vi "ClassNameCompare1.vi"(10 "NodeClass":string, 11 "classlist":string[](array[string])) -> (3 "match":bool)   [LabVIEW 2025, in "CEF.lvlib"]
doc: "Copyright 2017 National Instruments Corporation\n\nLicensed under the Apache License, Version 2.0 (the \"License\"); you may not use this file except in compliance with the License. You may obtain a copy of the License at http://www.apache.org/licenses/LICENSE-2.0\nUnless required by applicable law or agreed to in writing, software distributed under the License is distributed on an \"AS IS\" BASIS, WITHOUT WARRANTIES OR CONDITIONS OF ANY KIND, either express or implied. See the License for the specific language governing permissions and limitations under the License."
uses:
  CEF.lvlib
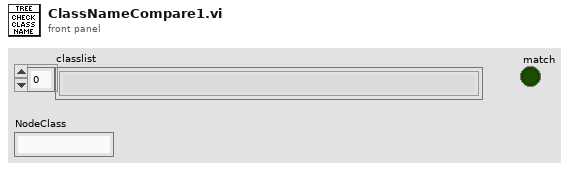
[diagram p1: front panel]
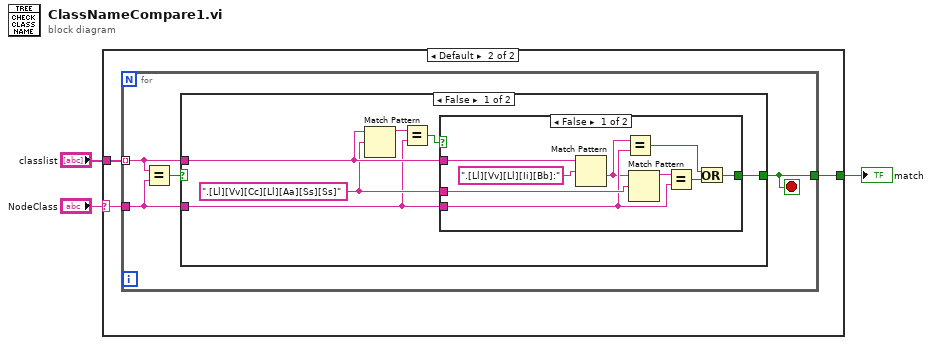
[diagram p0: block diagram]
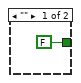
[diagram p2: hidden frame]
diagram:
  n1 = case shown="Default" "NodeClass" {
    selector: "NodeClass" -> [_ w5]
    tunnel: "classlist" -> [_ w7]
    tunnel: [FALSE w6] -> w2
    frame "" {
    }
    frame Default {
      n2 = for {
        tunnel: w7 -> [w9] mode=indexing
        tunnel: w5 -> [w8]
        tunnel: [w10] -> w6
        stop <- w10 stop-if-true
        n3 = Equal?(x=w9, y=w8) -> (x = y?=w11:bool)
        n4 = case shown="False" w11 {
          selector: w11 -> [_ w28]
          tunnel: [w15 w28] -> w10
          tunnel: w9 -> [w14 _]
          tunnel: w8 -> [w12 _]
          frame False {
            w13 = ".[Ll][Vv][Cc][Ll][Aa][Ss][Ss]" ("regular expression")
            n5 = Match Pattern(string=w14, regular expression=w13) -> (before substring=w17:string)  [unwired: 1 in, 3 out]
            n6 = Equal?(x=w17, y=w12) -> (x = y?=w16:bool)
            n7 = case shown="False" w16 {
              selector: w16 -> [_ w27]
              tunnel: [w21 w27] -> w15
              tunnel: w14 -> [w26 _]
              tunnel: w13 -> [w24 _]
              tunnel: w12 -> [w20 _]
              frame False {
                n8 = Match Pattern(string=w26, regular expression=".[Ll][Vv][Ll][Ii][Bb]:") -> (after substring=w18:string)  [unwired: 1 in, 3 out]
                n9 = Equal?(x=w18, y=w20) -> (x = y?=w23:bool)
                n10 = Match Pattern(string=w18, regular expression=w24) -> (before substring=w19:string)  [unwired: 1 in, 3 out]
                n11 = Equal?(x=w19, y=w20) -> (x = y?=w22:bool)
                n12 = Or(x=w23, y=w22) -> (x .or. y?=w21:bool)
              }
              frame True {
              }
            }
          }
          frame True {
          }
        }
      }
    }
  }
  "match" <- w2
